vi "serialize.ob.cmd.vi"(11 "OrderBook.Commands.in":T1[](array[typedef])=[{"type"=enum."AddOrder", "side"=66, "orderId "=48, "quantity"=20000, "symbol"=4702127773838221344, "price"=9050, "executed.qty"=0, "canceled.qty"=0, "remaining.qty"=0, "seconds"=0, "nanoseconds"=0, "Add"=FALSE, "Edit"=FALSE, "Remove"=FALSE}] {"symbol" format="%.0x"; "orderId" format="%.0x"; "side" format="%.0x"}) -> (3 "Words.Out":u64[](array[numeric])=[1, 66, 48, 20000, 4702127773838221344, 9050, 0, 0, 0, 0, 0, 0, 0, 0, 0, 0, 2, 66, 48, 0, 0, 9050, 200, 0, 0, 0, 0, 0, 0, 0, 0, 0, 5, 66, 48, 1400, 6076284164848492576, 9050, 0, 0, 0, 0, 0, 0, 0, 0, 0, 0] format="%.0x")   [LabVIEW 2020]
uses:
  fpga/common/orderbook.command.type.ctl
  fpga/common/orderbook.command.ctl
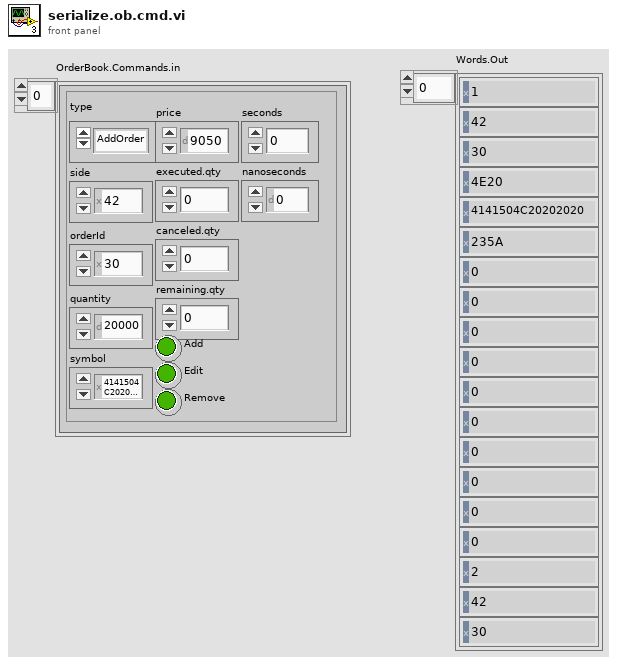
[diagram p1: front panel]
types:
  T1 = typedef "orderbook.command.ctl" = cluster{"type":T2, "side":u8, "orderId ":u64, "quantity":u32, "symbol":u64, "price":u64, "executed.qty":u32, "canceled.qty":u32, "remaining.qty":u32, "seconds":u64, "nanoseconds":u64, "Add":bool, "Edit":bool, "Remove":bool}
  T2 = typedef "orderbook.command.type.ctl" = enum8{"Time", "AddOrder", "OrderExecuted", "OrderExecutedAtPrice", "ReduceSize", "ModifyOrder", "DeleteOrder", "Get.Everything", "Get.All.Orders", "Get.Top"}
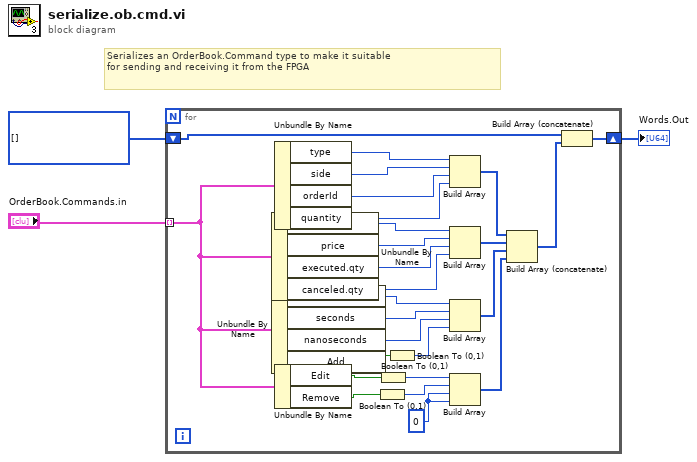
[diagram p0: block diagram]
diagram:
  # "Serializes an OrderBook.Command type to make it suitable\nfor sending and receiving it from the FPGA"
  n1 = for {
    tunnel: "OrderBook.Commands.in" -> [w8] mode=indexing
    shift-right: [w16] -> w1
    shift-left: u64[] [] -> [w18]
    w23 = u64 0 ("element")
    n2 = Unbundle By Name(w8) -> ("symbol"=w29:u64, "price"=w28:u64, "executed.qty"=w27:u32, "canceled.qty"=w26:u32)
    n3 = Unbundle By Name(w8) -> ("remaining.qty"=w25:u32, "seconds"=w24:u64, "nanoseconds"=w15:u64, "Add"=w14:bool)
    n4 = Unbundle By Name(w8) -> ("type"=w7:T2, "side"=w6:u8, "orderId"=w5:u64, "quantity"=w4:u32)
    n5 = Unbundle By Name(w8) -> ("Edit"=w11:bool, "Remove"=w12:bool)
    n6 = Boolean To (0,1)(Boolean=w12) -> (0, 1=w9:i16)
    n7 = Boolean To (0,1)(Boolean=w11) -> (0, 1=w10:i16)
    n8 = Boolean To (0,1)(Boolean=w14) -> (0, 1=w13:i16)
    n9 = Build Array(w7, w6, w5, w4) -> (w22:u64[])
    n10 = Build Array(w29, w28, w27, w26) -> (w21:u64[])
    n11 = Build Array(w25, w24, w15, w13) -> (w20:u64[])
    n12 = Build Array(w10, w9, w23, w23) -> (w19:u64[])
    n13 = Build Array (concatenate)(w22, w21, w20, w19) -> (w17:u64[])
    n14 = Build Array (concatenate)(w18, w17) -> (w16:u64[])
  }
  "Words.Out" <- w1
